vi "Create Attribute.vi"(8 "error in (no error)":errorcluster, 9 "Variant":variant, 10 "Label.Text":string, 11 "Refnum in":T1) -> (0 "error out":errorcluster, 3 "Refnum out":T1)   [LabVIEW 2019]
uses:
  <vilib>/UPVI/lvhdf5/library.llb/HDF5 Ref.ctl
  <vilib>/UPVI/lvhdf5/dataset.llb/LVH5D Operation.ctl
  <vilib>/UPVI/lvhdf5/dataset.llb/Simple OpenCreateReplace Dataset (Variant).vi
  <vilib>/UPVI/lvhdf5/dataset.llb/H5Dwrite (Variant).vi
  <vilib>/UPVI/lvhdf5/dataset.llb/Simple OpenCreateReplace Dataset.xnode
  <vilib>/UPVI/lvhdf5/dataset.llb/H5Dwrite.xnode
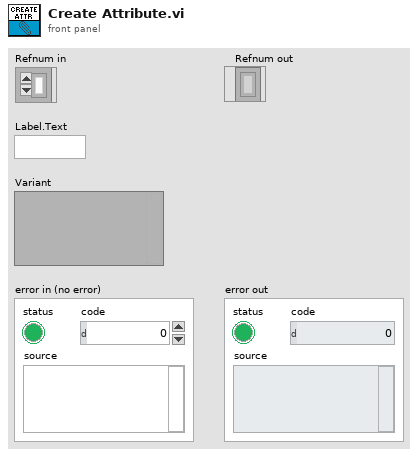
[diagram p1: front panel]
types:
  T1 = typedef "HDF5 Ref.ctl" = refnum<k1>
  T2 = typedef "LVH5D Operation.ctl" = enum16{"open", "replace", "create", "open or create", "create or replace", "create or replace with confirmation"}
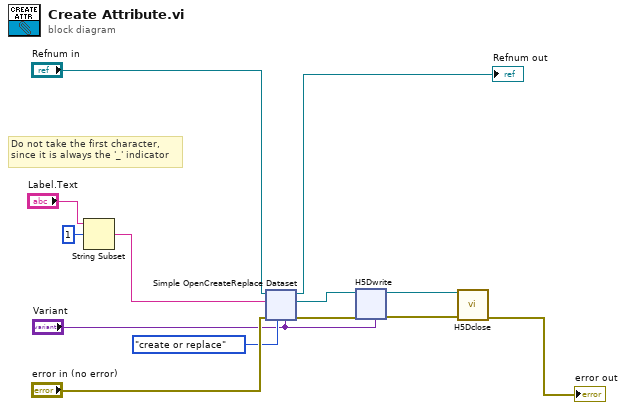
[diagram p0: block diagram]
diagram:
  # "Do not take the first character,\nsince it is always the '_' indicator"
  n1 = String Subset(string="Label.Text", offset (0)=1) -> (substring=w10:string)  [unwired: 1 in]
  n2 = xnode "Simple OpenCreateReplace Dataset"("Dataset Path"=w10, "HDF5 Ref"="Refnum in", "error in (no error)"="error in (no error)", "operation"=LVH5D_Operation."create or replace", "Datatype and Dataspace"="Variant") -> ("HDF5 Dataset Ref out"=w3:T1, "HDF5 Ref out"=→"Refnum out":T1, "error out"=w5:errorcluster)  [unwired: 3 in]
  n3 = xnode "H5Dwrite"("HDF5 Dataset Ref"=w3, "error in (no error)"=w5, "Data"="Variant") -> ("HDF5 Ref out"=w2:T1, "error out"=w4:errorcluster)  [unwired: 4 in]
  n4 = call <vilib>:"H5Dclose.vi"("error in (no error)"=w4, "HDF5 Dataset Ref"=w2) -> ("error out"=→"error out":errorcluster)  [unwired: 7 in]
